vi "Check Status No Objects.vi"(8 "error in (no error)":errorcluster) -> (0 "error out":errorcluster, 1 "Status":string, 2 "Ready?":bool)   [LabVIEW 2009]
doc: "Checks if the instrument is powered on and updates its member data with the instrument's current status."
uses:
  Tektronix AFG 3000 Series/Tektronix AFG 3000 Series.lvlib
  Tektronix AFG 3000 Series/controls.llb/Sweep Time Parameter.ctl
  Tektronix AFG 3000 Series/controls.llb/Sweep Frequency.ctl
  Tektronix AFG 3000 Series/controls.llb/Voltage.ctl
  Global/GPIB Numbers.vi
  Tektronix AFG 3000 Series/controls.llb/Waveform Shape.ctl
  Tektronix AFG 3000 Series/controls.llb/Sweep Spacing.ctl
  FG Channel Settings.ctl
panel:
  out "Output Cluster":T1
  in  "Input Cluster":T1
  in  "Channel Settings":T2={"General Settings"={" Frequency"=0.0, " Phase"=0.0, " Run Mode"=0, " Waveform Shape"=0, "Output on?"=FALSE}, "Voltage Settings"={"Amplitude"=0.0, "Offset"=0.0}, "Ramp Settings"={"Ramp Symmetry (%)"=50.0}, "Pulse Settings"={"Leading Edge Time "=5e-09, "Trailing Edge Time"=5e-09, "Duty Cycle (%)"=50.0}, "Sweep Mode Settings"={"Start Freq. "=0.0, "Stop Freq.  "=0.0, "Sweep spacing"=0, "Sweep time"=0.0, "Hold time"=0.0, "Return time"=0.0}, "Burst Mode Settings"={"Burst Mode "=1, "Burst Count"=5}, "AM Settings"={"AM Source "=0, "Modulation Waveform "=0, "Modulation Frequency "=1000.0, "Modulation Depth "=0.0}, "FM Settings"={"FM Source "=0, "Modulation Waveform "=0, "Modulation Frequency"=100.0, "Peak Deviation "=100.0}} {"General Settings"."Waveform Shape" items=["Sinusoid", "Square", "Pulse", "Ramp", "PRNoise", "DC", "SINC", "Gaussian", "Lorentz", "ERise", "EDecay", "Haversine", "User 1", "User 2", "User 3", "User 4", "EMemory", "EFile"]; "General Settings"."Run Mode" items=["Continuous", "AM", "FM", "PM", "FSK", "PWM", "Sweep", "Burst"]; "FM Settings"."Modulation Waveform" items=["Sine", "Square", "Triangle", "Ramp", "Down Ramp", "Noise", "User 1", "User 2", "User 3", "User 4", "EMEMory", "EFILe"]; "FM Settings"."FM Source" items=["Internal", "External"]; "AM Settings"."Modulation Waveform" items=["Sine", "Square", "Triangle", "Ramp", "Down Ramp", "Noise"]; "AM Settings"."AM Source" items=["Internal", "External"]; "Burst Mode Settings"."Burst Mode" items=["Triggered", "Gated"]; "Sweep Mode Settings"."Sweep spacing" items=["linear", "log"]; "Pulse Settings"."Trailing Edge Time" format="%#.6g"; "Pulse Settings"."Leading Edge Time" format="%#.6g"; "Ramp Settings"."Ramp Symmetry (%)" min=0.0 max=100.0 step=1.0 format="%.2f"}
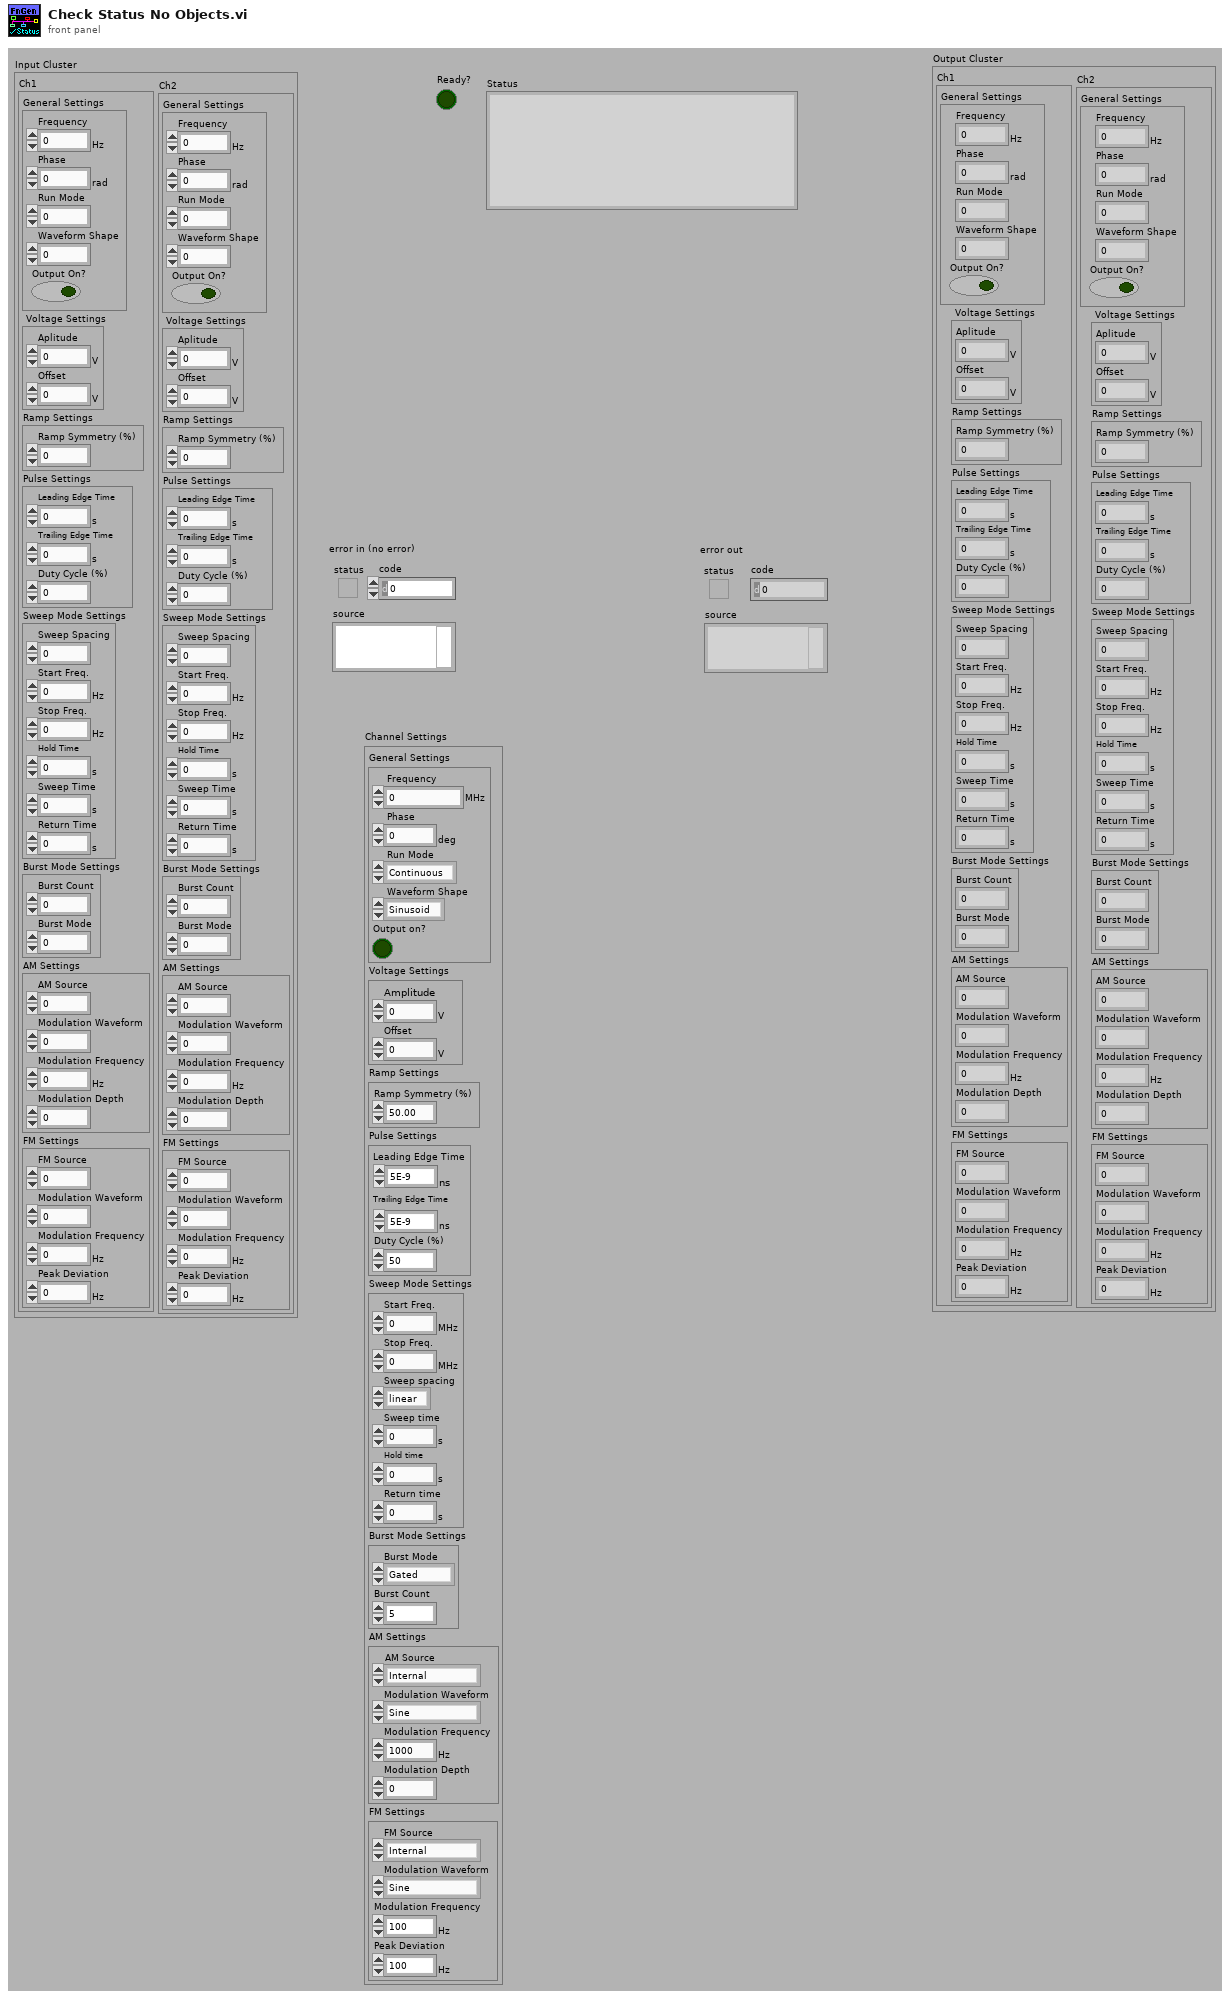
[diagram p1: front panel]
types:
  T1 = cluster{"Ch1":cluster{"General Settings":cluster{"Frequency":dbl[unit], "Phase":dbl[unit], "Run Mode":u16, "Waveform Shape":u16, "Output On?":bool}, " Voltage Settings":cluster{"Aplitude":dbl[unit], "Offset":dbl[unit]}, "Ramp Settings":cluster{"Ramp Symmetry (%)":dbl}, "Pulse Settings":cluster{"Leading Edge Time":dbl[unit], "Trailing Edge Time":dbl[unit], "Duty Cycle (%)":dbl}, "Sweep Mode Settings":cluster{"Sweep Spacing":u16, "Start Freq.":dbl[unit], "Stop Freq.":dbl[unit], "Hold Time":dbl[unit], "Sweep Time":dbl[unit], "Return Time":dbl[unit]}, "Burst Mode Settings":cluster{"Burst Count":i32, "Burst Mode":u16}, "AM Settings":cluster{"AM Source":u16, "Modulation Waveform":u16, "Modulation Frequency":dbl[unit], "Modulation Depth":dbl}, "FM Settings":cluster{"FM Source":u16, "Modulation Waveform":u16, "Modulation Frequency":dbl[unit], "Peak Deviation":dbl[unit]}}, "Ch2":cluster{"General Settings":cluster{"Frequency":dbl[unit], "Phase":dbl[unit], "Run Mode":u16, "Waveform Shape":u16, "Output On?":bool}, " Voltage Settings":cluster{"Aplitude":dbl[unit], "Offset":dbl[unit]}, "Ramp Settings":cluster{"Ramp Symmetry (%)":dbl}, "Pulse Settings":cluster{"Leading Edge Time":dbl[unit], "Trailing Edge Time":dbl[unit], "Duty Cycle (%)":dbl}, "Sweep Mode Settings":cluster{"Sweep Spacing":u16, "Start Freq.":dbl[unit], "Stop Freq.":dbl[unit], "Hold Time":dbl[unit], "Sweep Time":dbl[unit], "Return Time":dbl[unit]}, "Burst Mode Settings":cluster{"Burst Count":i32, "Burst Mode":u16}, "AM Settings":cluster{"AM Source":u16, "Modulation Waveform":u16, "Modulation Frequency":dbl[unit], "Modulation Depth":dbl}, "FM Settings":cluster{"FM Source":u16, "Modulation Waveform":u16, "Modulation Frequency":dbl[unit], "Peak Deviation":dbl[unit]}}}
  T2 = typedef "FG Channel Settings.ctl" = cluster{"General Settings":cluster{" Frequency":dbl[unit], " Phase":dbl[unit], " Run Mode":u16, " Waveform Shape":T3, "Output on?":bool}, "Voltage Settings":cluster{"Amplitude":dbl[unit], "Offset":dbl[unit]}, "Ramp Settings":cluster{"Ramp Symmetry (%)":dbl}, "Pulse Settings":cluster{"Leading Edge Time ":dbl[unit], "Trailing Edge Time":dbl[unit], "Duty Cycle (%)":dbl}, "Sweep Mode Settings":cluster{"Start Freq. ":dbl[unit], "Stop Freq.  ":dbl[unit], "Sweep spacing":T4, "Sweep time":dbl[unit], "Hold time":dbl[unit], "Return time":dbl[unit]}, "Burst Mode Settings":cluster{"Burst Mode ":u16, "Burst Count":i32}, "AM Settings":cluster{"AM Source ":u16, "Modulation Waveform ":u16, "Modulation Frequency ":dbl[unit], "Modulation Depth ":dbl}, "FM Settings":cluster{"FM Source ":u16, "Modulation Waveform ":u16, "Modulation Frequency":dbl[unit], "Peak Deviation ":dbl[unit]}}
  T3 = typedef "Waveform Shape.ctl" = u16
  T4 = typedef "Sweep Spacing.ctl" = u16
  T5 = typedef "GPIB Type Def.ctl" = cluster{"Name":string, "bus":dbl, "GPIB":dbl, "GPIB as string":string, "byte":i32, "VISA Resource Name":refnum<visa-resource-name>}
  T6 = typedef "Voltage.ctl" = enum16{"amplitude", "offset", "high", "low", "high limit", "low limit"}
  T7 = typedef "Sweep Frequency.ctl" = enum16{"center", "span", "start", "stop"}
  T8 = typedef "Sweep Time Parameter.ctl" = enum16{"sweep time", "hold time", "return time"}
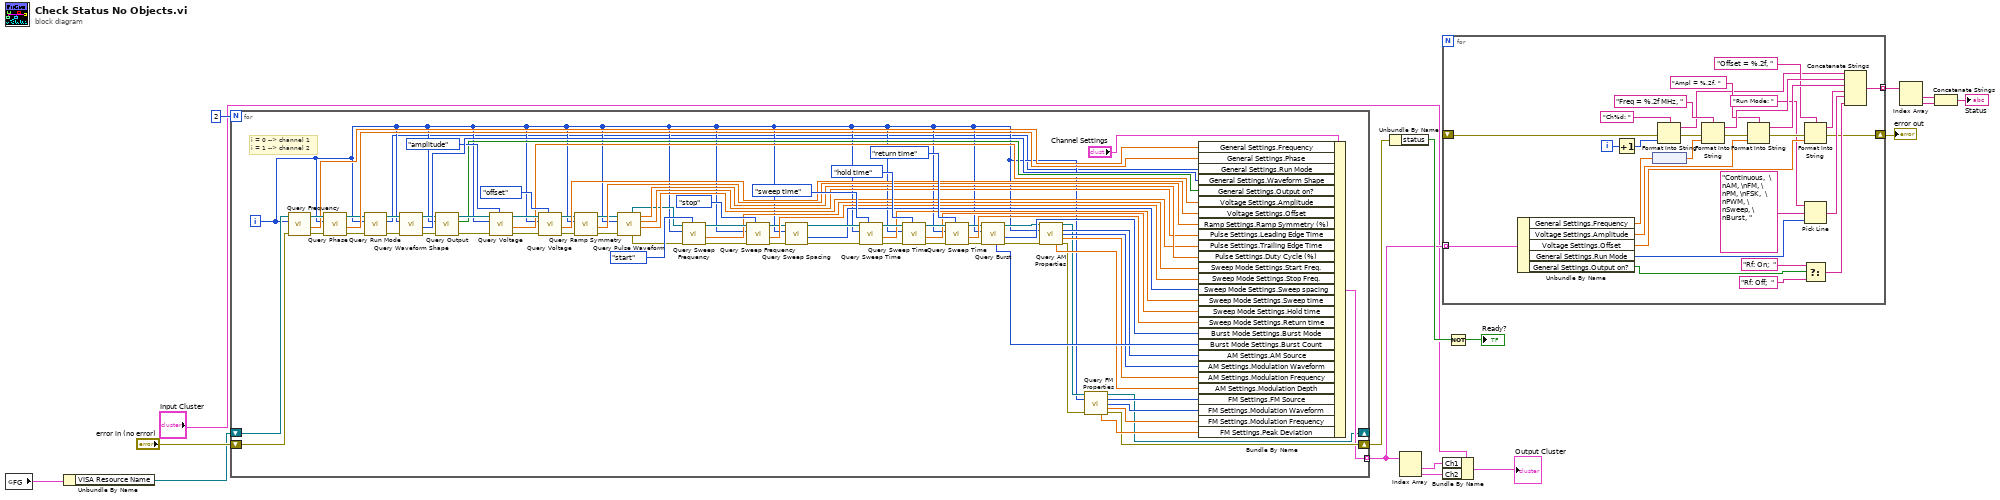
[diagram p0: block diagram]
diagram:
  n1 = global read "GPIB Numbers.vi" "FG"() -> (w6:T5)
  n2 = Unbundle By Name(w6) -> ("VISA Resource Name"=w5:refnum<visa-resource-name>)
  n3 = for {
    N: 2 -> [_]
    shift-right: [w33] -> w15
    shift-left: "error in (no error)" -> [w83]
    tunnel: [w32] -> w14 mode=indexing
    shift-right: [w31] -> _
    shift-left: w5 -> [w30]
    i -> [w19]
    # "i = 0 --> channel 1\ni = 1 --> channel 2"
    n4 = call "Query Frequency.vi"("error in (no error)"=w83, "Channel (0: Channel 1)"=w19, "VISA resource name"=w30) -> ("error out"=w82:errorcluster, "frequency"=w80:dbl[unit], "VISA resource name out"=w89:refnum<visa-resource-name>)  [unwired: 6 out]
    n5 = call "Query Phase.vi"("error in (no error)"=w82, "Channel (0: Channel 1)"=w19, "VISA resource name"=w89) -> ("error out"=w21:errorcluster, "phase"=w79:dbl[unit], "VISA resource name out"=w23:refnum<visa-resource-name>)  [unwired: 6 out]
    n6 = call "Query Run Mode.vi"("error in (no error)"=w21, "Channel (0: Channel 1)"=w19, "VISA resource name"=w23) -> ("error out"=w20:errorcluster, "Run Mode"=w18:u16, "VISA resource name out"=w22:refnum<visa-resource-name>)  [unwired: 6 out]
    n7 = call "Query Waveform Shape.vi"("error in (no error)"=w20, "Channel (0: Channel 1)"=w19, "VISA resource name"=w22) -> ("error out"=w26:errorcluster, "Waveform Shape"=w78:T3, "VISA resource name out"=w28:refnum<visa-resource-name>)  [unwired: 6 out]
    n8 = call "Query Output.vi"("error in (no error)"=w26, "Channel (0: Channel 1)"=w19, "VISA resource name"=w28) -> ("error out"=w25:errorcluster, "Output Enabled?"=w24:bool, "VISA resource name out"=w27:refnum<visa-resource-name>)  [unwired: 6 out]
    n9 = call "Query Voltage.vi"("Voltage Param (amplitude)"=Voltage."amplitude", "error in (no error)"=w25, "Channel (0: Channel 1)"=w19, "VISA resource name"=w27) -> ("error out"=w45:errorcluster, "voltage"=w29:dbl[unit], "VISA resource name out"=w75:refnum<visa-resource-name>)  [unwired: 5 out]
    n10 = call "Query Voltage.vi"("Voltage Param (amplitude)"=Voltage."offset", "error in (no error)"=w45, "Channel (0: Channel 1)"=w19, "VISA resource name"=w75) -> ("error out"=w44:errorcluster, "voltage"=w74:dbl[unit], "VISA resource name out"=w73:refnum<visa-resource-name>)  [unwired: 5 out]
    n11 = call "Query Ramp Symmetry.vi"("error in (no error)"=w44, "Channel (0: Channel 1)"=w19, "VISA resource name"=w73) -> ("error out"=w43:errorcluster, "Symmetry (%)"=w72:dbl, "VISA resource name out"=w71:refnum<visa-resource-name>)  [unwired: 6 out]
    n12 = call "Query Pulse Waveform.vi"("error in (no error)"=w43, "Channel (0: Channel 1)"=w19, "VISA resource name"=w71) -> ("Trailing"=w68:dbl[unit], "Leading"=w69:dbl[unit], "Duty Cycle"=w70:dbl, "error out"=w42:errorcluster, "VISA resource name out"=w67:refnum<visa-resource-name>)  [unwired: 4 out]
    n13 = call "Query Sweep Frequency.vi"("Sweep Frequency"=Sweep_Frequency."start", "error in (no error)"=w42, "Channel (0: Channel 1)"=w19, "VISA resource name"=w67) -> ("error out"=w41:errorcluster, "frequency"=w66:dbl[unit], "VISA resource name out"=w92:refnum<visa-resource-name>)  [unwired: 5 out]
    n14 = call "Query Sweep Frequency.vi"("Sweep Frequency"=Sweep_Frequency."stop", "error in (no error)"=w41, "Channel (0: Channel 1)"=w19, "VISA resource name"=w92) -> ("error out"=w40:errorcluster, "frequency"=w65:dbl[unit], "VISA resource name out"=w64:refnum<visa-resource-name>)  [unwired: 5 out]
    n15 = call "Query Sweep Spacing.vi"("error in (no error)"=w40, "Channel (0: Channel 1)"=w19, "VISA resource name"=w64) -> ("error out"=w39:errorcluster, "Sweep spacing (linear)"=w62:T4, "VISA resource name out"=w63:refnum<visa-resource-name>)  [unwired: 6 out]
    n16 = call "Query Sweep Time.vi"("Sweep Time Param (sweep time)"=Sweep_Time_Parameter."sweep time", "error in (no error)"=w39, "Channel (0: Channel 1)"=w19, "VISA resource name"=w63) -> ("error out"=w38:errorcluster, "time"=w61:dbl[unit], "VISA resource name out"=w90:refnum<visa-resource-name>)  [unwired: 5 out]
    n17 = call "Query Sweep Time.vi"("Sweep Time Param (sweep time)"=Sweep_Time_Parameter."hold time", "error in (no error)"=w38, "Channel (0: Channel 1)"=w19, "VISA resource name"=w90) -> ("error out"=w37:errorcluster, "time"=w60:dbl[unit], "VISA resource name out"=w91:refnum<visa-resource-name>)  [unwired: 5 out]
    n18 = call "Query Sweep Time.vi"("Sweep Time Param (sweep time)"=Sweep_Time_Parameter."return time", "error in (no error)"=w37, "Channel (0: Channel 1)"=w19, "VISA resource name"=w91) -> ("error out"=w36:errorcluster, "time"=w59:dbl[unit], "VISA resource name out"=w58:refnum<visa-resource-name>)  [unwired: 5 out]
    n19 = call "Query Burst.vi"("error in (no error)"=w36, "Channel (0: Channel 1)"=w19, "VISA resource name"=w58) -> ("error out"=w35:errorcluster, "Burst Mode"=w57:u16, "VISA resource name out"=w55:refnum<visa-resource-name>, "Burst Count"=w56:i32)  [unwired: 5 out]
    n20 = call "Query AM Properties.vi"("VISA resource name"=w55, "Channel (0: Channel 1)"=w19, "error in (no error)"=w35) -> ("VISA resource name out"=w50:refnum<visa-resource-name>, "AM Source"=w54:u16, "Modulation Waveform"=w53:u16, "Modulation Frequency"=w52:dbl[unit], "Modulation Depth"=w51:dbl, "error out"=w34:errorcluster)  [unwired: 7 out]
    n21 = call "Query FM Properties.vi"("VISA resource name"=w50, "Channel (0: Channel 1)"=w19, "error in (no error)"=w34) -> ("VISA resource name out"=w31:refnum<visa-resource-name>, "FM Source"=w49:u16, "Modulation Waveform"=w48:u16, "Modulation Frequency"=w47:dbl[unit], "Peak Deviation"=w46:dbl[unit], "error out"=w33:errorcluster)  [unwired: 7 out]
    n22 = Bundle By Name(cluster="Channel Settings", "General Settings.Frequency"=w80, "General Settings.Phase"=w79, "General Settings.Run Mode"=w18, "General Settings.Waveform Shape"=w78, "General Settings.Output on?"=w24, "Voltage Settings.Amplitude"=w29, "Voltage Settings.Offset"=w74, "Ramp Settings.Ramp Symmetry (%)"=w72, "Pulse Settings.Leading Edge Time"=w69, "Pulse Settings.Trailing Edge Time"=w68, "Pulse Settings.Duty Cycle (%)"=w70, "Sweep Mode Settings.Start Freq."=w66, "Sweep Mode Settings.Stop Freq."=w65, "Sweep Mode Settings.Sweep spacing"=w62, "Sweep Mode Settings.Sweep time"=w61, "Sweep Mode Settings.Hold time"=w60, "Sweep Mode Settings.Return time"=w59, "Burst Mode Settings.Burst Mode"=w57, "Burst Mode Settings.Burst Count"=w56, "AM Settings.AM Source"=w54, "AM Settings.Modulation Waveform"=w53, "AM Settings.Modulation Frequency"=w52, "AM Settings.Modulation Depth"=w51, "FM Settings.FM Source"=w49, "FM Settings.Modulation Waveform"=w48, "FM Settings.Modulation Frequency"=w47, "FM Settings.Peak Deviation"=w46) -> (w32:T2)
  }
  n23 = Unbundle By Name(w15) -> ("status"=w17:bool)
  n24 = Index Array(array=w14) -> (element #1=w3:T2, element #2=w2:T2)  [unwired: 2 in]
  n25 = for {
    tunnel: w14 -> [w104] mode=indexing
    shift-right: [w98] -> w13
    shift-left: _ -> [w97]
    tunnel: [w96] -> w12 mode=indexing
    i -> [w103]
    n26 = Unbundle By Name(w104) -> ("General Settings.Frequency"=w121:dbl[unit], "Voltage Settings.Amplitude"=w119:dbl[unit], "Voltage Settings.Offset"=w118:dbl[unit], "General Settings.Run Mode"=w117:u16, "General Settings.Output on?"=w116:bool)
    n27 = Increment(x=w103) -> (x+1=w93:i32)
    n28 = node(w121) -> (w120:dbl)
    n29 = Format Into String(format string="Ch%d: " ("string (\"\")"), error in=w97, w93) -> (resulting string=w95:string, error out=w101:errorcluster)  [unwired: 1 in]
    n30 = Format Into String(format string="Freq = %.2f MHz, " ("string (\"\")"), error in=w101, w120) -> (resulting string=w112:string, error out=w100:errorcluster)  [unwired: 1 in]
    n31 = Format Into String(format string="Ampl = %.2f, " ("string (\"\")"), error in=w100, w119) -> (resulting string=w109:string, error out=w99:errorcluster)  [unwired: 1 in]
    n32 = Format Into String(format string="Offset = %.2f, " ("string (\"\")"), error in=w99, w118) -> (resulting string=w107:string, error out=w98:errorcluster)  [unwired: 1 in]
    n33 = Pick Line(string ("")="Run Mode: ", multi-line string="Continuous,  \nAM, \nFM, \nPM, \nFSK,  \nPWM, \nSweep, \nBurst, ", line index=w117) -> (output string=w105:string)
    n34 = Select(t="Rf: On;  " ("string (\"\")"), s=w116, f="Rf: Off;  " ("string (\"\")")) -> (s? t:f=w106:string)
    n35 = Concatenate Strings(w95, w112, w109, w107, w105, w106) -> (w96:string)
  }
  "error out" <- w13
  n36 = Bundle By Name(cluster="Input Cluster", "Ch1"=w3, "Ch2"=w2) -> (→"Output Cluster":T1)
  n37 = Not(x=w17) -> (.not. x?=→"Ready?":bool)
  n38 = Index Array(array=w12) -> (element #1=w11:string, element #2=w10:string)  [unwired: 2 in]
  n39 = Concatenate Strings(w11, w10) -> (→"Status":string)
